vi "get_concatenate_node_term.vi"(0 "Terms[] In":refnum<vi>[](array[refnum]), 11 "error in (no error)":errorcluster) -> (4 "Terms[]  Out":refnum<vi>[](array[refnum]), 8 "Concantenate Term":refnum<vi>, 15 "error out":errorcluster)   [LabVIEW 2018]
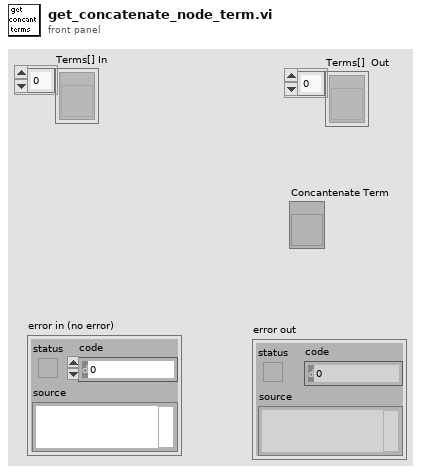
[diagram p1: front panel]
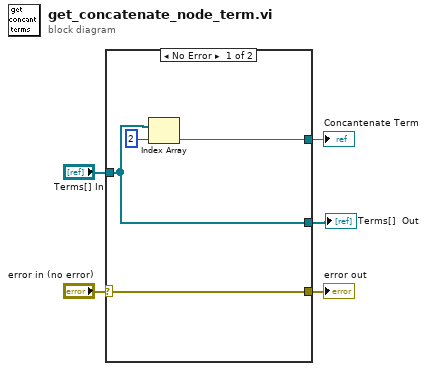
[diagram p0: block diagram]
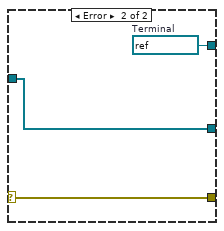
[diagram p2: hidden frame]
diagram:
  n1 = case shown="No Error" "error in (no error)" {
    selector: "error in (no error)" -> [w7 w12]
    tunnel: "Terms[] In" -> [w6 w11]
    tunnel: [w8 w10] -> w4
    tunnel: [w7 w12] -> w2
    tunnel: [w6 w11] -> w1
    frame No Error {
      n2 = Index Array(array=w6, index=2) -> (element=w8:refnum<vi>)
    }
    frame Error {
      w10 = refnum<vi> refnum  # Terminal
    }
  }
  "Concantenate Term" <- w4
  "error out" <- w2
  "Terms[]  Out" <- w1
